vi "Substration.vi"(8 "error in (no error)":errorcluster, 10 "Input2":string="71.772763E+0", 11 "Input1":string="71.772763E+0") -> (0 "error out":errorcluster, 3 "In1 - In2":string)   [LabVIEW 2012]
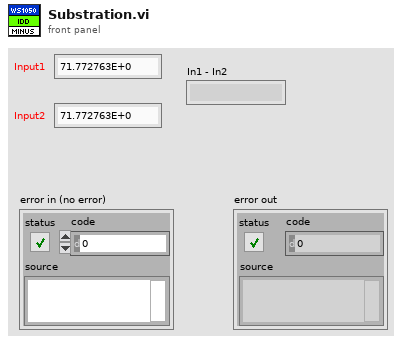
[diagram p1: front panel]
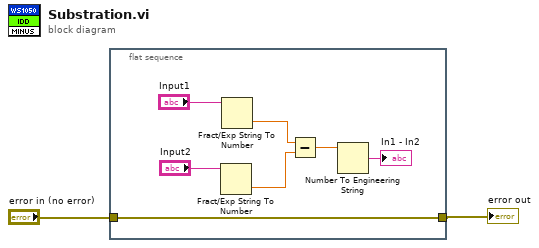
[diagram p0: block diagram]
diagram:
  n1 = flat-sequence {
    tunnel: "error in (no error)" -> [w3]
    tunnel: [w3] -> w1
    frame #0 {
      n2 = Fract/Exp String To Number(string="Input2") -> (number=w6:dbl)  [unwired: 3 in, 1 out]
      n3 = Fract/Exp String To Number(string="Input1") -> (number=w7:dbl)  [unwired: 3 in, 1 out]
      n4 = Subtract(x=w7, y=w6) -> (x-y=w5:dbl)
      n5 = Number To Engineering String(4:w5) -> (0:→"In1 - In2":string)  [unwired: 3 in]
    }
  }
  "error out" <- w1
